vi "Systematic Error Correction.vi"() -> ()   [LabVIEW 2013]
panel:
  out "Результат измерений":string
  out "Поправка":dbl
  in  "Знаков после запятой":dbl=3.0
  in  "Отн. погр. вн":dbl(slide) min=0.0 max=5.0 step=0.25 scale=0.0..5.0
  in  "Выбор вольтметра":bool
  out "Абс. инстр. погрешность, В":dbl
  out "Показания вольтметра, В":dbl
  in  "Сопротивление источника, Ом":dbl
  in  "Напряжение ИП":T1(ring)
  out "Шкала вольтметра, В":dbl(knob) scale=0.0..1.573
  in  "Выбор предела\nV-SIM1":i32(knob)=8 min=0 max=8 step=1 scale=0.0..8.0
  # "Вычисление и исключение систематической погрешности"
  # "V-SIM2"
  # "V-SIM1"
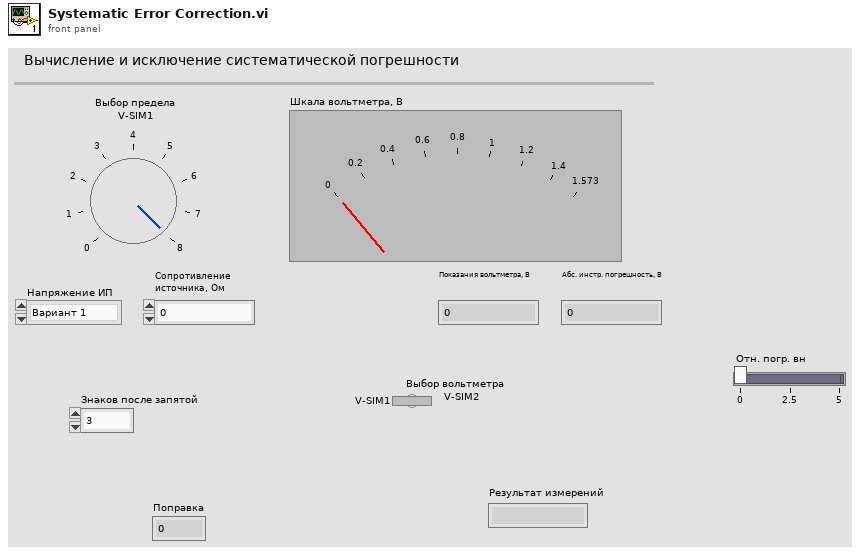
[diagram p1: front panel]
types:
  T1 = enum16{"Вариант 1", "Вариант 2", "Вариант 3", "Вариант 4", "Вариант 5", "Вариант 6", "Вариант 7", "Вариант 8", "Вариант 9", "Вариант 10", "Вариант 11", "Вариант 12"}
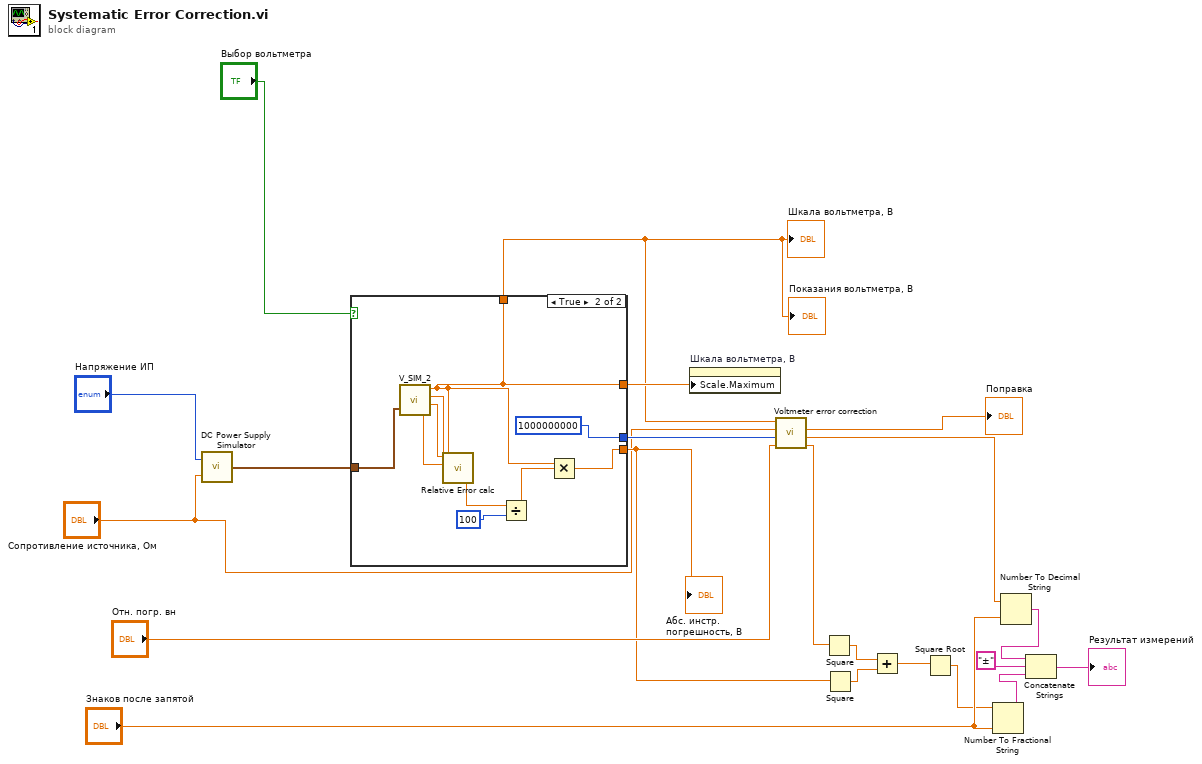
[diagram p0: block diagram]
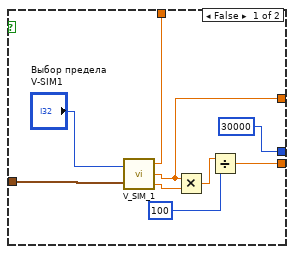
[diagram p2: hidden frame]
diagram:
  n1 = call "DC Power Supply Simulator.vi"("Rвн, Ом"="Сопротивление источника, Ом", "Напряжение ИП"="Напряжение ИП") -> ("Выход"=w20:cluster{"Uип, В":dbl, "Rвн_д, Ом":dbl})
  n2 = case shown="True" "Выбор вольтметра" {
    tunnel: w20 -> [w30 w37]
    tunnel: [w27 w36] -> w13
    tunnel: [w26 w35] -> w19
    tunnel: [w25 w35] -> w17
    tunnel: [30000 1000000000] -> w16
    frame False {
      n3 = call "V_SIM_1.vi"("Выбор предела измерений"="Выбор предела\nV-SIM1", "Вход"=w30) -> ("Показания вольтметра, В"=w25:dbl, "Установленный предел, В"=w26:dbl, "Класс точности (привед. погр.), %"=w28:dbl)
      n4 = Multiply(x=w26, y=w28) -> (x*y=w24:dbl)
      n5 = Divide(x=w24, y=100) -> (x/y=w27:dbl)
    }
    frame True {
      n6 = call "V_SIM_2.vi"("Вход"=w37) -> ("Показания вольтметра, В"=w35:dbl, "Установленный предел, В"=w38:dbl, "c"=w40:dbl, "d"=w39:dbl)  [unwired: 1 in]
      n7 = call "Relative Error calc.vi"("X"=w38, "Xk"=w35, "d"=w39, "c"=w40) -> ("Относительная погрешность, %"=w33:dbl)
      n8 = Divide(x=w33, y=100) -> (x/y=w32:dbl)
      n9 = Multiply(x=w35, y=w32) -> (x*y=w36:dbl)
    }
  }
  "Шкала вольтметра, В" <- w17
  "Показания вольтметра, В" <- w17
  "Абс. инстр. погрешность, В" <- w13
  n10 = property on="Шкала вольтметра, В" class="Knob (strict)"("Scale.Maximum"=w19) -> ()  [unwired: 2 in, 2 out]
  n11 = call "Voltmeter error correction.vi"("Относителоьная погрешность определения Rвн, %"="Отн. погр. вн", "Rвх вольтметра , Ом"=w16, "Rвн источинка, Ом"="Сопротивление источника, Ом", "Показания вольтметра , В"=w17) -> ("Неисключенная методическая погрешность , В"=w14:dbl, "Исправленные показания , В"=w6:dbl, "Поправка , В"=→"Поправка":dbl)  [unwired: 1 out]
  n12 = Square(x=w14) -> (x^2=w12:dbl)
  n13 = Square(x=w13) -> (x^2=w11:dbl)
  n14 = Add(x=w12, y=w11) -> (x+y=w10:dbl)
  n15 = Square Root(x=w10) -> (sqrt(x)=w4:dbl)
  n16 = Number To Fractional String(number=w4, precision (6)="Знаков после запятой") -> (F-format string=w9:string)  [unwired: 2 in]
  n17 = Number To Decimal String(number=w6, width (-)="Знаков после запятой") -> (decimal integer string=w7:string)
  n18 = Concatenate Strings(w7, "±", w9) -> (→"Результат измерений":string)
